vi "Restore sequence from multiple images.vi"(6 "Milliseconds per frame":dbl format="%.2f", 7 "error in":errorcluster, 9 "Sequence files handle":T1, 10 "Directory path":path) -> (0 "error out":errorcluster, 3 "Last frame number written out":u32)   [LabVIEW 2011]
doc: "Takes a sequence of individual image files (e.g., TIFFs) or a SEQ file and loads it in to an acquisition file.\n\nINPUTS:\nDirectory name (sequence name with path). If left empty, the program will prompt for name.\nSequence of images.\nFile format (AIPD as default)"
uses:
  Sequence files handle.ctt
  Seq file v 1/Offset table.ctl
  Seq file v 1/Offset.ctl
  Seq file v 1/file number.ctl
  Header2 file data.ctl
panel:
  out "Pixel depth":u32(ring) items=["8 bits", "16 bits", "Float", "Complex", "RGB", "HSL"]
  out "File data type":u32(ring) items=["1 bit", "2 bits", "4 bits", "8 bits", "16 bits (unsigned)", "16 bits (signed)", "16 bits (RGB chunky)", "24 bits (RGB chunky)", "24 bits (RGB planar)", "32 bits (unsigned)", "32 bits (signed)", "32 bits (RGB chunky)", "32 bits (float)", "48 bits (Complex 2x24 int)", "64 bits (Complex 2x32 float)", "32 bits (HSL)"]
  out "Extension":string
  out "Prefix":string
  out "file number":string
  out "file name":string
  out "Path":path
  in  "Quit":bool
  out "Frame number":i32
  out "File":path
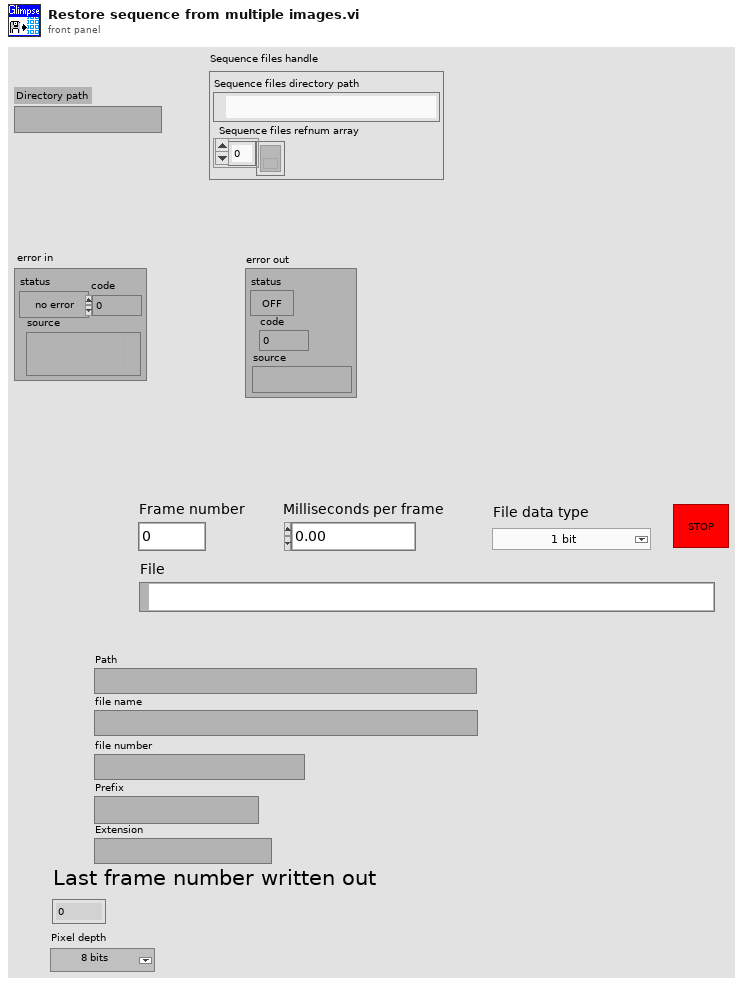
[diagram p1: front panel]
types:
  T1 = typedef "Sequence files handle.ctt" = cluster{"Sequence files directory path":path, "Sequence files refnum array":refnum<file>[]}
  T2 = enum32{"existing file", "new file", "new or existing file", "existing dir", "new dir", "new or existing dir", "existing file (use LLBs)", "new file (use LLBs)", "new or existing file (use LLBs)", "new or existing file or directory (use LLBs)"}
  T3 = typedef "Offset table.ctl" = cluster{"offset":T4, "file number":T5}[]
  T4 = typedef "Offset.ctl" = i32
  T5 = typedef "file number.ctl" = u8
  T6 = cluster{"stripped path":path, string, string, i32}
  T7 = typedef "Image Type" = u32
  T8 = typedef "IMAQ Image.ctl" = refnum<image>
  T9 = typedef "Header2 file data.ctl" = cluster{"Camera":string, "Microscope":string, "Microscope software version":string, "Laser names":string[], "Filter names":string[], "Lasers array":u16[][], "Filter array":u16[], "Flow rate array":dbl[], "Temperature array":dbl[], "Field array":u16[], "Is header2 info present?":bool, "Description Info":string, "Stage xyz array":dbl[][]}
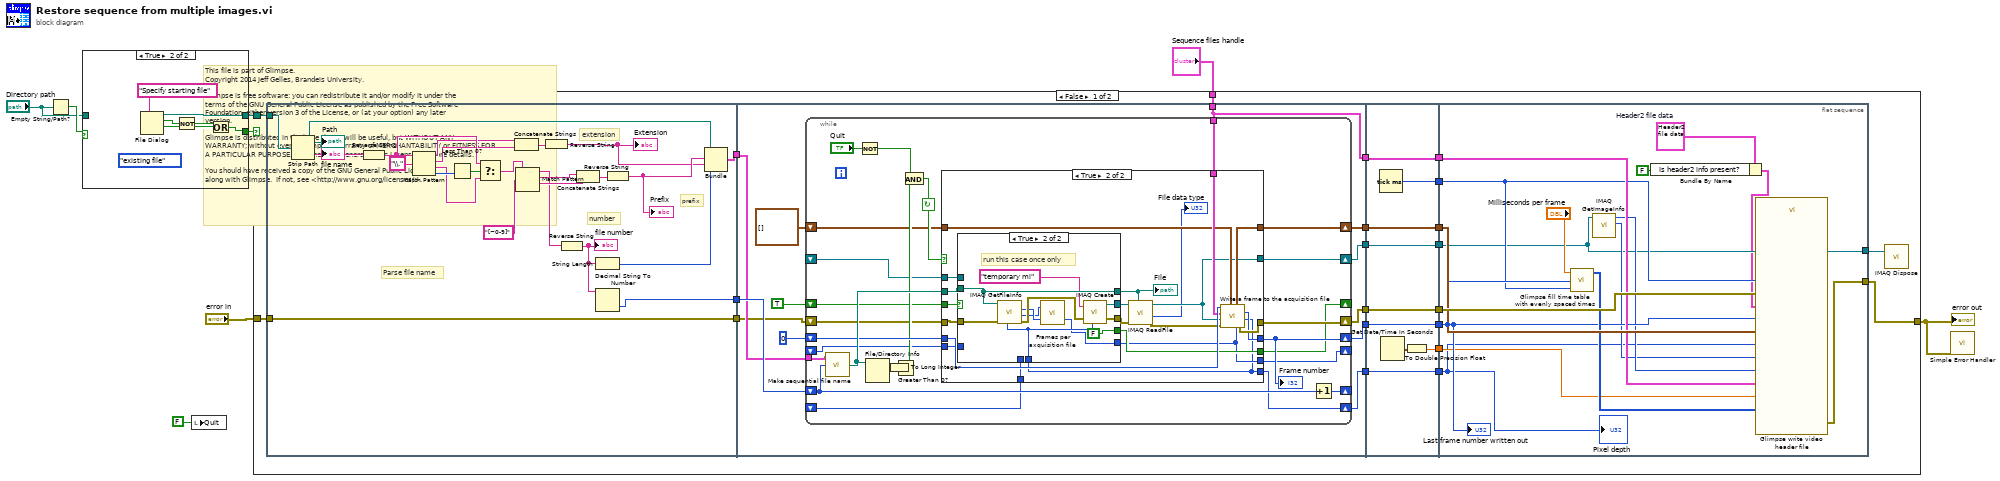
[diagram p0: block diagram]
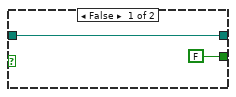
[diagram p5: hidden frame]
diagram:
  # "This file is part of Glimpse. \nCopyright 2014 Jeff Gelles, Brandeis University.    \n\nGlimpse is free software: you can redistribute it and/or modify it under the \nterms of the GNU General Public License as published by the Free Software \nFoundation, either version 3 of the License, or (at your option) any later \nversion.\n\nGlimpse is distributed in the hope that it will be useful, but WITHOUT ANY \nWARRANTY; without even the implied warranty of MERCHANTABILITY or FITNESS FOR \nA PARTICULAR PURPOSE.  See the GNU General Public License for more details.\n\nYou should have received a copy of the GNU General Public License\nalong with Glimpse.  If not, see <http://www.gnu.org/licenses/>."
  n1 = Empty String/Path?(string/path="Directory path") -> (empty?=w8:bool)
  n2 = case shown="True" w8 {
    tunnel: [w10 w16] -> w6
    tunnel: "Directory path" -> [w10 _]
    tunnel: [FALSE ("cancelled") w11] -> w5
    frame False {
    }
    frame True {
      (unwired) T2."existing file" ("select mode (2)")
      n3 = File Dialog(7:"Specify starting file" ("prompt")) -> (1:w12:bool, 2:w14:bool, 3:w16:path)  [unwired: 1 in, 6 out]
      n4 = Not(x=w14) -> (.not. x?=w13:bool)
      n5 = Or(x=w13, y=w12) -> (x .or. y?=w11:bool)
    }
  }
  n6 = local write "Quit"(FALSE ("Quit")) -> ()
  n7 = case shown="False" w5 {
    tunnel: w6 -> [w38 _]
    tunnel: "error in" -> [w37 w170]
    tunnel: [w36 w170] -> w2
    tunnel: "Sequence files handle" -> [w20 _]
    frame False {
      n8 = flat-sequence {
        tunnel: w38 -> [w62]
        tunnel: w37 -> [w39]
        tunnel: [w39] -> w35
        tunnel: [w40] -> w34
        tunnel: [w41] -> w33
        tunnel: w35 -> [w72]
        tunnel: [w63] -> w32
        tunnel: [w64] -> w31
        tunnel: w34 -> [w73]
        tunnel: w33 -> [w74]
        tunnel: [w70] -> w30
        tunnel: [w67] -> w29
        tunnel: [w69] -> w28
        tunnel: [w65] -> w27
        tunnel: w20 -> [w63]
        tunnel: w32 -> [w149]
        tunnel: [w149] -> w26
        tunnel: w31 -> [w148]
        tunnel: [w148] -> w25
        tunnel: w30 -> [w153]
        tunnel: [w153] -> w24
        tunnel: w29 -> [w152]
        tunnel: [w152] -> w23
        tunnel: w28 -> [w147]
        tunnel: [w147] -> w22
        tunnel: w27 -> [w151]
        tunnel: [w151] -> w21
        tunnel: [w146] -> w19
        tunnel: [w145] -> w18
        tunnel: [w168] -> w36
        tunnel: w26 -> [w166]
        tunnel: w25 -> [w158]
        tunnel: w24 -> [w163]
        tunnel: w23 -> [w167]
        tunnel: w22 -> [w169]
        tunnel: w21 -> [w157]
        tunnel: w19 -> [w162]
        tunnel: w18 -> [w159]
        tunnel: [w157] -> w17
        frame #0 {
          # "number"
          # "prefix"
          # "extension"
          # "Parse file name"
          n9 = Strip Path(path=w62) -> (stripped path=w45:path, name=w61:string)
          "Path" <- w45
          "file name" <- w61
          n10 = Reverse String(1:w61) -> (0:w57:string)
          n11 = Match Pattern(string=w57, regular expression="\\.") -> (before substring=w55:string, match substring=w54:string, after substring=w56:string, offset past match=w59:i32)  [unwired: 1 out]
          n12 = Less Than 0?(x=w59) -> (x < 0?=w58:bool)
          n13 = Select(t=w57, s=w58, f=w56) -> (s? t:f=w52:string)
          n14 = Concatenate Strings(w55, w54) -> (w51:string)
          n15 = Match Pattern(string=w52, regular expression="[~0-9]") -> (before substring=w47:string, match substring=w49:string, after substring=w48:string)  [unwired: 2 out]
          n16 = Reverse String(1:w51) -> (0:w43:string)
          "Extension" <- w43
          n17 = Reverse String(1:w47) -> (0:w46:string)
          "file number" <- w46
          n18 = Concatenate Strings(w49, w48) -> (w50:string)
          n19 = String Length(string=w46) -> (length=w42:i32)
          n20 = Decimal String To Number(string=w46) -> (number=w41:i32)  [unwired: 3 out]
          n21 = Reverse String(1:w50) -> (0:w44:string)
          "Prefix" <- w44
          n22 = Bundle("stripped path"=w45, w44, w43, w42) -> (w40:T6)  [unwired: 1 out]
        }
        frame #1 {
          n23 = while {
            shift-left: 0 -> [w90]
            shift-right: [w89] -> w70
            shift-left: w72 -> [w87]
            shift-right: [w91] -> w69
            tunnel: w73 -> [w97]
            shift-left: w74 -> [w98]
            shift-right: [w99] -> _
            tunnel: w63 -> [w86]
            shift-right: [w84] -> w67
            shift-left: T3 [] ("Offset table out") -> [w85]
            shift-right: [w82] -> _
            shift-left: TRUE -> [w83]
            shift-right: [w81] -> w65
            shift-left: _ -> [w80]
            shift-right: [w79] -> w64
            shift-left: _ -> [w78]
            shift-right: [w77] -> _
            shift-left: _ -> [w76]
            stop <- w92 continue-if-true
            n24 = call "Make sequential file name.vi"("Serial number"=w98, "File name information"=w97) -> ("Path out"=w95:path)  [unwired: 1 in]
            n25 = Not(x="Quit") -> (.not. x?=w93:bool)
            n26 = File/Directory Info(path=w95) -> (size=w75:i64)  [unwired: 1 in, 6 out]
            n27 = To Long Integer(number=w75) -> (32bit integer=w96:i32)
            n28 = Greater Than 0?(x=w96) -> (x > 0?=w88:bool)
            n29 = And(x=w93, y=w88) -> (x .and. y?=w92:bool)
            n30 = case shown="True" w92 {
              tunnel: w95 -> [_ w116]
              tunnel: [w105 w127] -> w91
              tunnel: w90 -> [w106 w126]
              tunnel: [w106 w123] -> w89
              tunnel: w87 -> [w105 w117]
              tunnel: w86 -> [_ w125]
              tunnel: w85 -> [w104 w122]
              tunnel: [w104 w121] -> w84
              tunnel: [w102 w120] -> w81
              tunnel: w83 -> [w103 w119]
              tunnel: [w103 w118] -> w82
              tunnel: w80 -> [w102 w112]
              tunnel: [w101 w107] -> w79
              tunnel: w78 -> [w101 w110]
              tunnel: [w100 w109] -> w77
              tunnel: w76 -> [w100 w108]
              frame False {
              }
              frame True {
                n31 = case shown="True" w119 {
                  selector: w119 -> [w133 _]
                  tunnel: [w133 FALSE] -> w118
                  tunnel: w117 -> [w131 w143]
                  tunnel: w116 -> [w132 w142]
                  tunnel: [w132 w142] -> w115
                  tunnel: [w131 w139] -> w114
                  tunnel: [w130 w138] -> w113
                  tunnel: w112 -> [w130 _]
                  tunnel: [w129 w137] -> w107
                  tunnel: w110 -> [w129 _]
                  tunnel: [w128 w134] -> w109
                  tunnel: w108 -> [w128 _]
                  frame False {
                  }
                  frame True {
                    # "run this case once only"
                    n32 = call "IMAQ GetFileInfo"("error in (no error)"=w143, "File Path"=w142) -> ("error out"=w141:errorcluster, "Y Resolution"=w135:i32, "X Resolution"=w136:i32, "Image Type"=w137:T7)  [unwired: 6 out]
                    n33 = call "Frames per axquisition file.vi"("Output frame width"=w136, "Output frame height"=w135) -> ("Frames per acquisition file"=w134:i32)  [unwired: 1 out]
                    n34 = call "IMAQ Create"("Image Name"="temporary mi", "Image Type"=w137, "error in (no error)"=w141) -> ("New Image"=w138:T8, "error out"=w139:errorcluster)  [unwired: 1 in, 1 out]
                  }
                }
                "File" <- w115
                n35 = call "IMAQ ReadFile"("File Path"=w115, "error in (no error)"=w114, "Image"=w113) -> ("error out"=w124:errorcluster, "File Data Type out"=→"File data type":i32, "Image Out"=w120:T8)  [unwired: 2 in, 4 out]
                n36 = call "Write a frame to the acquisition file.vi"("Pixel depth"=w107, "Frames per acquisition file"=w109, "Offset table in"=w122, "error in"=w124, "Image In"=w120, "Sequence files handle"=w125, "Last frame number written in"=w126) -> ("error out"=w127:errorcluster, "Last frame number written out"=w123:u32, "Offset table out"=w121:T3)  [unwired: 2 out]
              }
            }
            "Frame number" <- w89
            n37 = Increment(x=w98) -> (x+1=w99:i32)
          }
        }
        frame #2 {
          n38 = Tick Count (ms)() -> (millisecond timer value=w146:u32)
          n39 = Get Date/Time In Seconds() -> (seconds since 1Jan1904=w150:timestamp)
          n40 = To Double Precision Float(number=w150) -> (double precision float=w145:dbl)
        }
        frame #3 {
          w156 = T9 {"Camera"="", "Microscope"="", "Microscope software version"="", "Laser names"=[], "Filter names"=[], "Lasers array"=[], "Filter array"=[], "Flow rate array"=[], "Temperature array"=[], "Field array"=[], "Is header2 info present?"=FALSE, "Description Info"="", "Stage xyz array"=[]}  # Header2 file data
          n41 = call "Glimpse fill time table with evenly spaced times.vi"("Element 0 of TTB"=w162, "Number of frames in sequence"=w163, "Milliseconds per frame"="Milliseconds per frame") -> ("TTB Array"=w165:u32[])  [unwired: 2 out]
          n42 = call "IMAQ GetImageInfo"("Image"=w157) -> ("Y Resolution"=w160:i32, "X Resolution"=w161:i32)  [unwired: 1 in, 8 out]
          n43 = Bundle By Name(cluster=w156, "Is header2 info present?"=FALSE) -> (w154:T9)
          n44 = call "Glimpse write video header file.vi"("Number of frames"=w163, "Sequence files handle"=w166, "Pixel depth\n(0=8 bit; 1= 16 bit)"=w158, "error in"=w169, "TTB Array"=w165, "Offsets Array"=w167, "Header2 file data"=w154, "Region width"=w161, "Region height"=w160, "Element 0 of TTB"=w162, "time of 1st frame, \nsec since 1/1/04"=w159) -> ("error out"=w168:errorcluster)  [unwired: 8 in]
          "Last frame number written out" <- w163
          "Pixel depth" <- w158
        }
      }
      n45 = call "IMAQ Dispose"("Image"=w17) -> ()  [unwired: 2 in, 4 out]
    }
    frame True {
    }
  }
  "error out" <- w2
  n46 = call <vilib>:"Simple Error Handler.vi"("error in (no error)"=w2) -> ()  [unwired: 1 in, 8 out]
